vi "Header file compatibility manager.vi"() -> (0 "ROI file format version":i32, 1 "[ROI Time (us)]":dbl[](array[numeric]), 2 "Z-Stack Header data":T1={"Number of POI"=0, "Number of Miniscans"=0, "Number of Trials"=0, "Number of Cycles "=0, "# Averaged Frames"=0, "Laser power (%)"=0, "Pockels"=0.0, "Acquisition Length (sec)"=0.0, "Fill time (us)"=0.0, "DwellTime (us)"=0.0, "Miniscan Dwell time per pixel (us)"=0.0, "PMT 1"=0.0, "PMT 2"=0.0, "Back Apperture"=0.0, "Zoom"=0.0, "Number of Pixels in Miniscan"=0, "Frame Size"=200, "Field of View"=0.0, "X centre"=0.0, "Y centre"=0.0, "AOL Z"=0.0} {"Frame Size" items=["100X100"=100, "128X128"=128, "200X200"=200, "256X256"=256, "512X512"=512, "1024x1024"=1024, "2048x2048"=2048]; "Back Apperture" format="%#.6g"; "Pockels" format="%#.6g"; "PMT 2" format="%#.6g"; "PMT 1" format="%#.6g"; "Miniscan Dwell time per pixel (us)" format="%#.6g"; "Zoom" format="%#.6g"; "DwellTime (us)" format="%#.6g"; "Acquisition Length (sec)" format="%#.6g"; "Fill time (us)" format="%#.6g"}, 3 "[Pixels in ROI]":i32[](array[numeric]))   [LabVIEW 2013]
uses:
  Experiment header interface/Typedefs/Header parameters cluster-Zstack.ctl
  Typedefs/Frame Size.ctl
  Typedefs/Get-Set-Clear Control.ctl
  Experiment header interface/Typedefs/Header file interface module functions enum.ctl
  Global Variables/General Globals.vi
panel:
  # "Zstack header parameters"
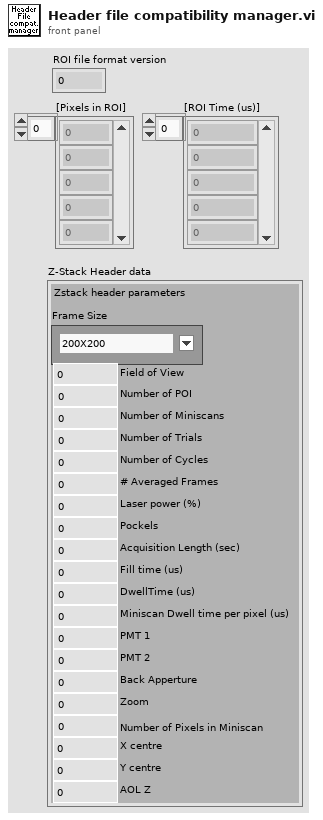
[diagram p1: front panel]
types:
  T1 = typedef "Header parameters cluster-Zstack.ctl" = cluster{"Number of POI":u16, "Number of Miniscans":u16, "Number of Trials":u16, "Number of Cycles ":u16, "# Averaged Frames":u16, "Laser power (%)":u8, "Pockels":dbl, "Acquisition Length (sec)":dbl, "Fill time (us)":dbl, "DwellTime (us)":dbl, "Miniscan Dwell time per pixel (us)":dbl, "PMT 1":dbl, "PMT 2":dbl, "Back Apperture":dbl, "Zoom":dbl, "Number of Pixels in Miniscan":u16, "Frame Size":T2, "Field of View":dbl, "X centre":dbl, "Y centre":dbl, "AOL Z":dbl}
  T2 = typedef "Frame Size.ctl" = u16
  T3 = typedef "Header file interface module functions enum.ctl" = enum16{"Load experiment header file", "Save experiment header file", "Clear stored values", "Read stored values", "Update specific value in memory", "Update all values in memory"}
  T4 = typedef "Get-Set-Clear Control.ctl" = enum16{"Get", "Set", "Clear"}
  T5 = typedef "Functional Parameters Cluster.ctl" = cluster{"ROI data":dbl[][], "ROI format version":i32, "Norm ROI data":dbl[][], "Norm. ROI format version":i32, "Z norm":dbl[], "Z norm format version":i32}
  T6 = typedef "Header parameters cluster-ALL.ctl" = cluster{"Imaging Protocol":T7, "Number of POI":u16, "Number of Miniscans":u16, "Number of Trials":u16, "Number of Cycles ":u64, "# Averaged Frames":u16, "Laser power (%)":u8, "Pockels":dbl, "Acquisition Length (sec)":dbl, "Fill time (us)":dbl, "POI Dwell time (us)":dbl, "Miniscan Dwell time per pixel (us)":dbl, "PMT 1":dbl, "PMT 2":dbl, "Back Apperture":dbl, "Zoom":dbl, "Frame Size":T2, "Center Frequency":dbl, "Field of View":dbl, "DwellTime (us)":dbl, "Wavelength (nm)":dbl, "AOL Z":dbl, "AOL Mode":T8, "GridXY":dbl, "GridZ":dbl, "TriggerDelay (sec)":dbl, "Number of Pixels in Miniscan":u16, "Experiment folder path":path, "X centre":dbl, "Y centre":dbl, "Angle (degrees)":dbl, "Plane Mode":T9, "Software version":dbl, "Objective":T10, "MotorZ Calibration":u32, "Pockels Calibration":u32, "Threshold":u16[], "Video length (sec)":dbl, "Frame rate (fps)":u8, "Rectangle ROI length (pixels)":u16, "Rectangle ROI height (pixels)":u16}
  T7 = typedef "Imaging Protocols enum.ctl" = enum16{"AOL Z-Stack", "Motor Z Stack", "Functional Acquisition", "Single Plane Acquisition", "Volume Acquisition", "Live Imaging", "Live Plane Imaging", "Live Volume Imaging"}
  T8 = typedef "AOL modes.ctl" = enum16{"Raster", "Structural", "Pointing", "Mini Scan", "Alignment"}
  T9 = typedef "Plane Mode.ctl" = u16
  T10 = typedef "Objective selector control enum.ctl" = string
  T11 = typedef "ROI file columns mapping.ctl" = cluster{"\"ROI index\" column index":i32, "\"ROI ID\" column index":i32, "\"ROI Time (ns)\" column index":i32, "\"Pixels in ROI\" column index":i32, "\"X (X start)\" column index":i32, "\"Y (Y start)\" column index":i32, "\"Z (Z start)\" column index":i32, "\"X (X stop)\" column index":i32, "\"Y (Y stop)\" column index":i32, "\"Z (Z stop)\" column index":i32, "\"Angle (deg)\" column index":i32, "Composite ID":i32, "Number of lines":i32, "Frame Size":i32, "Zoom":i32, "Laser Power (%)":i32, "ROI group ID":i32}
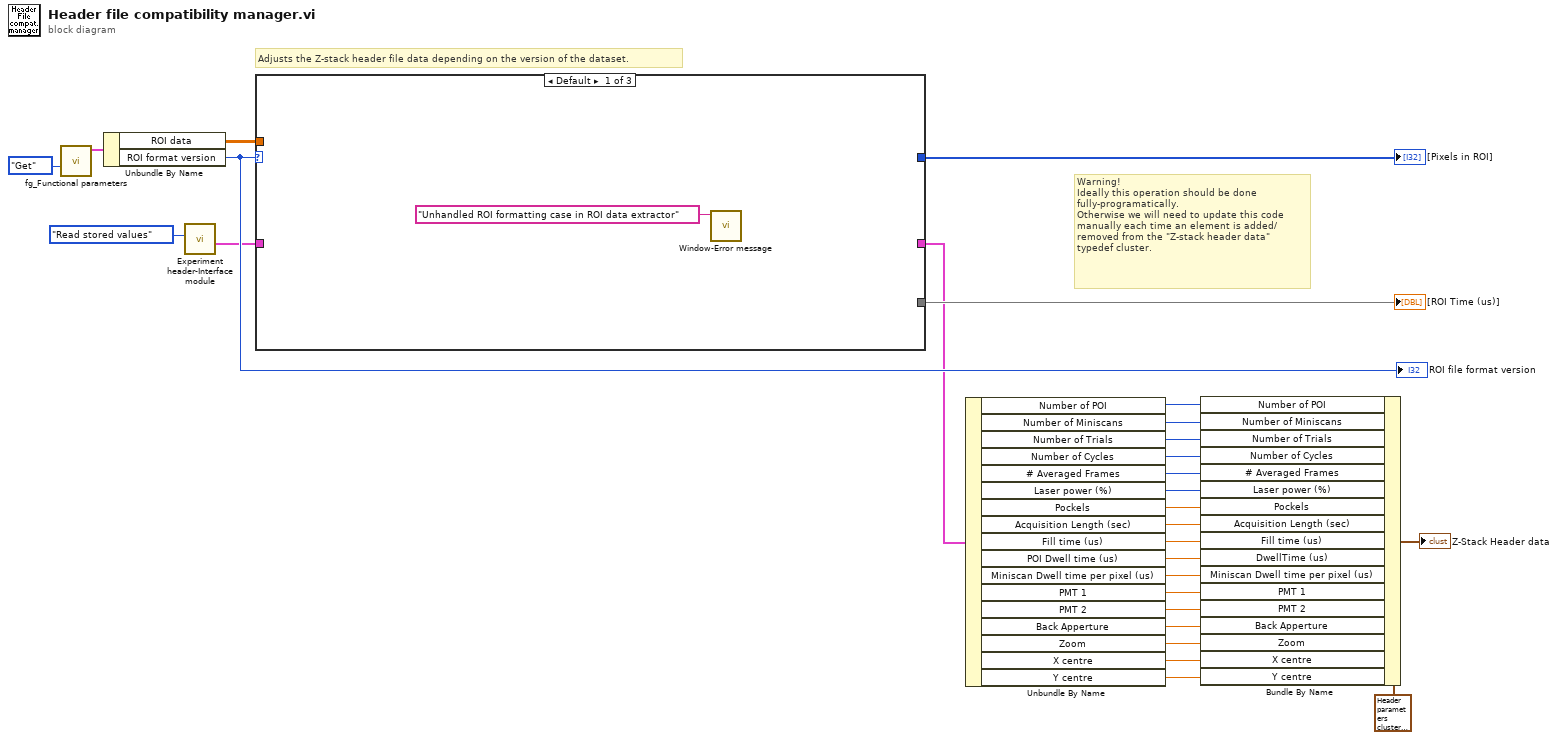
[diagram p0: block diagram]
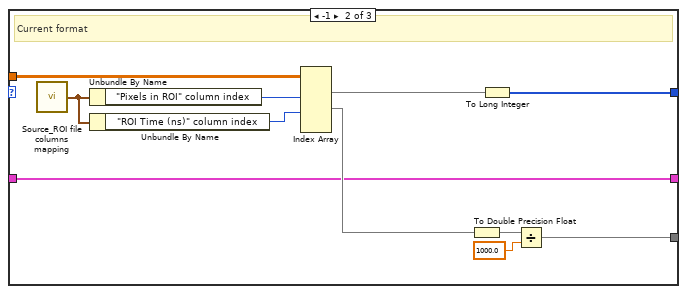
[diagram p2: hidden frame]
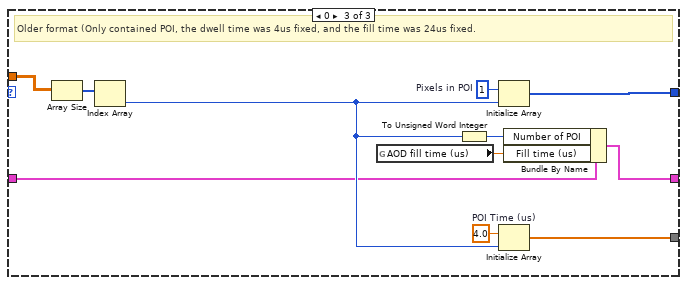
[diagram p3: hidden frame]
diagram:
  # "Warning!\nIdeally this operation should be done fully-programatically.\nOtherwise we will need to update this code manually each time an element is added/removed from the \"Z-stack header data\" typedef cluster."
  # "Adjusts the Z-stack header file data depending on the version of the dataset."
  n1 = call "fg_Functional parameters.vi"("Function"=Get-Set-Clear_Control."Get") -> ("Functional Parameters"=w24:T5)  [unwired: 7 in, 3 out]
  n2 = Unbundle By Name(w24) -> ("ROI data"=w26:dbl[][], "ROI format version"=w23:i32)
  "ROI file format version" <- w23
  n3 = call "Experiment header-Interface module.vi"("Function"=Header_file_interface_module_functions_enum."Read stored values") -> ("All header parameters out"=w21:T6)  [unwired: 9 in, 1 out]
  n4 = case shown="Default" w23 {
    tunnel: w26 -> [_ w39 w51]
    tunnel: [_ w37 w44] -> w27
    tunnel: [_ w31 w46] -> w28
    tunnel: [_ w30 w49] -> w3
    tunnel: w21 -> [_ w30 w42]
    frame Default {
      n5 = call "Window-Error message.vi"("Message"="Unhandled ROI formatting case in ROI data extractor" ("message")) -> ()  [unwired: 10 in, 1 out]
    }
    frame -1 {
      # "Current format"
      n6 = call "Source_ROI file columns mapping.vi"() -> ("ROI file columns mapping"=w32:T11)  [unwired: 1 in]
      n7 = Unbundle By Name(w32) -> ("\"Pixels in ROI\" column index"=w38:i32)
      n8 = Unbundle By Name(w32) -> ("\"ROI Time (ns)\" column index"=w36:i32)
      n9 = Index Array(array=w39, index (col) #1=w38, index (col) #2=w36) -> (element #1=w40:dbl[], element #2=w33:dbl[])  [unwired: 4 in, 1 out]
      n10 = To Double Precision Float(number=w33) -> (double precision float=w34:dbl[])
      n11 = To Long Integer(number=w40) -> (32bit integer=w37:i32[])
      n12 = Divide(x=w34, y=1000.0) -> (x/y=w31:dbl[])
    }
    frame 0 {
      w45 = 1  # Pixels in POI
      w47 = 4.0  # POI Time (us)
      # "Older format (Only contained POI, the dwell time was 4us fixed, and the fill time was 24us fixed."
      n13 = Array Size(array=w51) -> (size(s)=w50:i32[])
      n14 = Index Array(array=w50) -> (element=w43:i32)  [unwired: 1 in]
      n15 = global read "General Globals.vi" "AOD fill time (us)"() -> (w41:dbl)
      n16 = To Unsigned Word Integer(number=w43) -> (unsigned 16bit integer=w48:u16)
      n17 = Initialize Array(w45, w43) -> (w44:i32[])
      n18 = Initialize Array(w47, w43) -> (w46:dbl[])
      n19 = Bundle By Name(cluster=w42, "Number of POI"=w48, "Fill time (us)"=w41) -> (w49:T6)
    }
  }
  "[ROI Time (us)]" <- w28
  "[Pixels in ROI]" <- w27
  n20 = Unbundle By Name(w3) -> ("Number of POI"=w19:u16, "Number of Miniscans"=w18:u16, "Number of Trials"=w17:u16, "Number of Cycles"=w16:u64, "# Averaged Frames"=w15:u16, "Laser power (%)"=w14:u8, "Pockels"=w13:dbl, "Acquisition Length (sec)"=w12:dbl, "Fill time (us)"=w11:dbl, "POI Dwell time (us)"=w10:dbl, "Miniscan Dwell time per pixel (us)"=w9:dbl, "PMT 1"=w8:dbl, "PMT 2"=w7:dbl, "Back Apperture"=w6:dbl, "Zoom"=w5:dbl, "X centre"=w2:dbl, "Y centre"=w1:dbl)
  n21 = Bundle By Name(cluster=T1 {"Number of POI"=0, "Number of Miniscans"=0, "Number of Trials"=0, "Number of Cycles "=0, "# Averaged Frames"=0, "Laser power (%)"=0, "Pockels"=0.0, "Acquisition Length (sec)"=0.0, "Fill time (us)"=0.0, "DwellTime (us)"=0.0, "Miniscan Dwell time per pixel (us)"=0.0, "PMT 1"=0.0, "PMT 2"=0.0, "Back Apperture"=0.0, "Zoom"=0.0, "Number of Pixels in Miniscan"=0, "Frame Size"=0, "Field of View"=0.0, "X centre"=0.0, "Y centre"=0.0, "AOL Z"=0.0} ("Z-Stack Header data"), "Number of POI"=w19, "Number of Miniscans"=w18, "Number of Trials"=w17, "Number of Cycles"=w16, "# Averaged Frames"=w15, "Laser power (%)"=w14, "Pockels"=w13, "Acquisition Length (sec)"=w12, "Fill time (us)"=w11, "DwellTime (us)"=w10, "Miniscan Dwell time per pixel (us)"=w9, "PMT 1"=w8, "PMT 2"=w7, "Back Apperture"=w6, "Zoom"=w5, "X centre"=w2, "Y centre"=w1) -> (→"Z-Stack Header data":T1)
